vi "Mean_fr_NaN_data.vi"(1 "Data":dbl[](array[numeric]) format="%.2f") -> (0 "Mean value":dbl format="%.2f")   [LabVIEW 2010]
uses:
  <vilib>/Analysis/NI_AALBase.lvlib
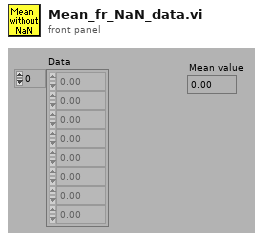
[diagram p1: front panel]
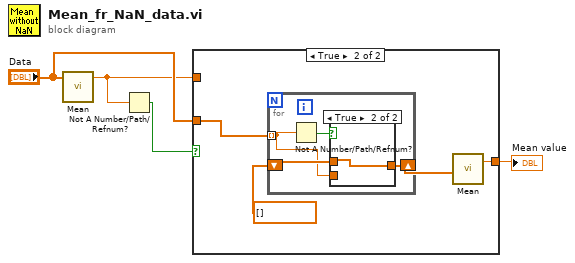
[diagram p0: block diagram]
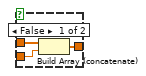
[diagram p3: hidden frame]
diagram:
  n1 = call <vilib>:"Mean.vi"("X"="Data") -> ("mean"=w2:dbl)  [unwired: 1 out]
  n2 = Not A Number/Path/Refnum?(number/path/refnum=w2) -> (NaN/Path/Refnum?=w1:bool)
  n3 = case shown="True" w1 {
    tunnel: "Data" -> [_ w9]
    tunnel: [w5 w7] -> w3
    tunnel: w2 -> [w5 _]
    frame False {
    }
    frame True {
      n4 = for {
        tunnel: w9 -> [w10] mode=indexing
        shift-right: [w12] -> w8
        shift-left: dbl[] [] -> [w13]
        n5 = Not A Number/Path/Refnum?(number/path/refnum=w10) -> (NaN/Path/Refnum?=w11:bool)
        n6 = case shown="True" w11 {
          tunnel: w13 -> [w16 w17]
          tunnel: [w15 w17] -> w12
          tunnel: w10 -> [w14 _]
          frame False {
            n7 = Build Array (concatenate)(w16, w14) -> (w15:dbl[])
          }
          frame True {
          }
        }
      }
      n8 = call <vilib>:"Mean.vi"("X"=w8) -> ("mean"=w7:dbl)  [unwired: 1 out]
    }
  }
  "Mean value" <- w3
